vi "ConfigureGausFitGuess (SubVI).vi"(10 "Array":dbl[](array[numeric]), 11 "Fitted Circle":T1) -> (3 "initial guess out":T2)   [LabVIEW 2016]
panel:
  in  "initial guess in":T2={"initial amplitude"=nan, "initial center"=nan, "initial standard deviation"=nan, "offset"=nan}
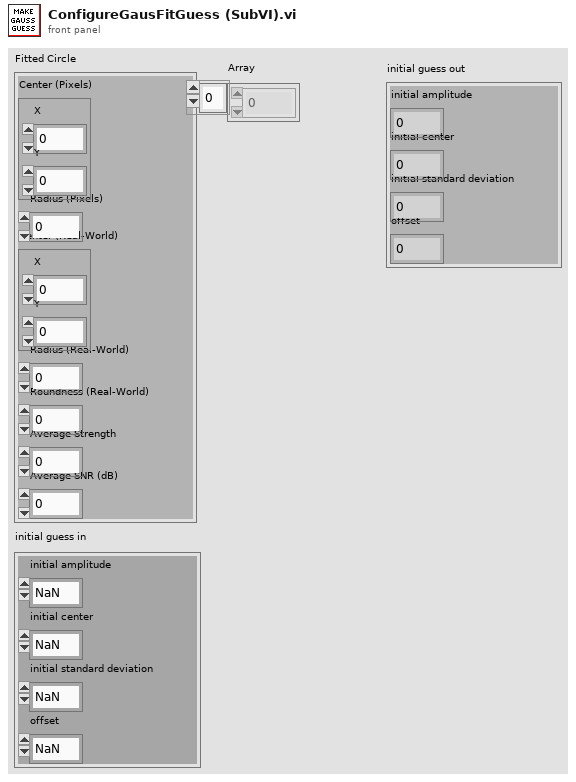
[diagram p1: front panel]
types:
  T1 = cluster{"Center (Pixels)":cluster{"X":sgl, "Y":sgl}, "Radius (Pixels)":dbl, "Center (Real-World)":cluster{"X":sgl, "Y":sgl}, "Radius (Real-World)":dbl, "Roundness (Real-World)":dbl, "Average Strength":dbl, "Average SNR (dB)":dbl}
  T2 = cluster{"initial amplitude":dbl, "initial center":dbl, "initial standard deviation":dbl, "offset":dbl}
  T3 = cluster{dbl, "Radius (Pixels)":dbl, "initial standard deviation":dbl, "offset":dbl}
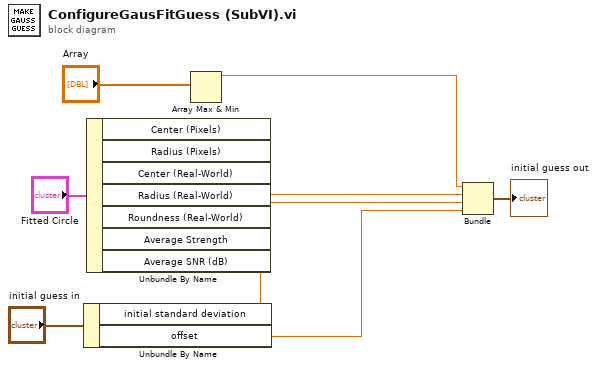
[diagram p0: block diagram]
diagram:
  n1 = Unbundle By Name("initial guess in") -> ("initial standard deviation"=w2:dbl, "offset"=w1:dbl)
  n2 = Unbundle By Name("Fitted Circle") -> ("Radius (Pixels)"=w4:dbl)  [unwired: 6 out]
  n3 = Array Max & Min(array="Array") -> (max value=w5:dbl)  [unwired: 3 out]
  n4 = Bundle(w5, "Radius (Pixels)"=w4, "initial standard deviation"=w2, "offset"=w1) -> (→"initial guess out":T3)  [unwired: 1 in]
